vi "Continuous DO Output.vi"() -> ()   [LabVIEW 2016]
uses:
  <vilib>/ULx/Create Channel.llb/ULx Create Channel (AI-Voltage-Basic).vi
  <vilib>/ULx/Timing.llb/ULx Timing (Sample Clock).vi
  <vilib>/ULx/Read.llb/ULx Read (Analog 1D Wfm NChan NSamp).vi
  <vilib>/Waveform/WDTOps.llb/WDT Index Channel DBL.vi
panel:
  in  "Boolean 3":bool
  out "Waveform Graph":dbl[](graph)
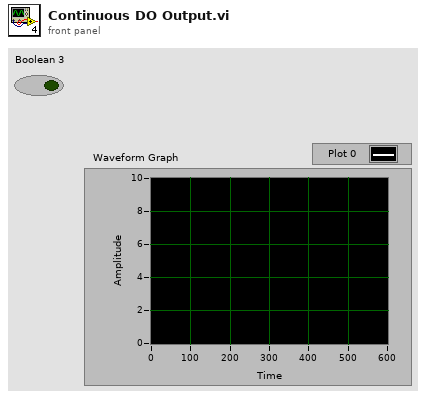
[diagram p1: front panel]
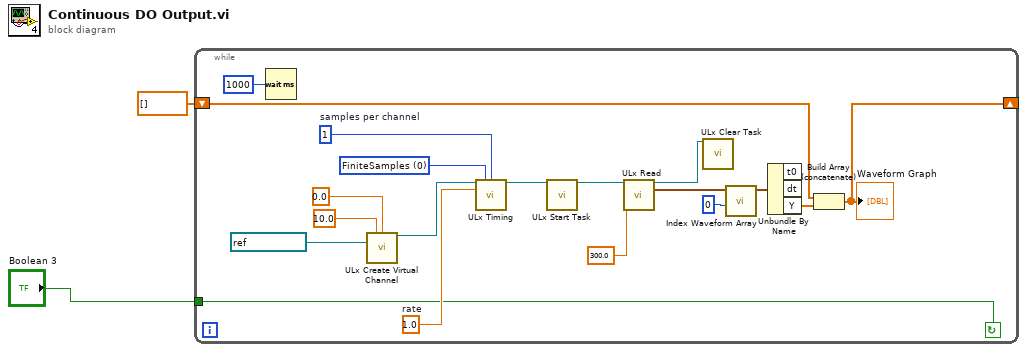
[diagram p0: block diagram]
diagram:
  n1 = while {
    shift-right: [w5] -> _
    shift-left: dbl[] [] -> [w7]
    tunnel: "Boolean 3" -> [w3]
    stop <- w3 continue-if-true
    w6 = 1  # samples per channel
    w17 = 0 items=["FiniteSamples", "ContinuousSamples"] ("sample mode")
    w16 = 1.0  # rate
    n2 = Wait (ms)(milliseconds to wait=u32 1000) -> ()  [unwired: 1 out]
    n3 = call-poly <vilib>:"ULx Create Virtual Channel.vi"("maximum value"=10.0, "minimum value"=0.0, "physical channels"=refnum<k21> "Dev0/Ai0" ("Test 1")) -> ("task out"=w14:refnum<k24>)  [unwired: 11 in, 1 out]
    n4 = call-poly <vilib>:"ULx Timing.vi"("task in"=w14, "sample mode"=w17, "samples per channel"=w6, "rate"=w16) -> ("task out"=w15:refnum<k24>)  [unwired: 10 in, 1 out]
    n5 = call <vilib>:"ULx Start Task.vi"("task in"=w15) -> ("task out"=w18:refnum<k24>)  [unwired: 13 in, 1 out]
    n6 = call-poly <vilib>:"ULx Read.vi"("task in"=w18, "timeout"=300.0) -> ("task out"=w11:refnum<k24>, "data"=w21:waveform(dbl)[])  [unwired: 11 in, 1 out]
    n7 = call <vilib>:"ULx Clear Task.vi"("task in"=w11) -> ()  [unwired: 14 in, 1 out]
    n8 = call-poly <vilib>:"Index Waveform Array.vi"("index"=0, "waveform array"=w21) -> ("waveform"=w20:waveform(dbl))  [unwired: 8 in, 1 out]
    n9 = Unbundle By Name(w20) -> ("Y"=w9:dbl[])  [unwired: 2 out]
    n10 = Build Array (concatenate)(w7, w9) -> (w5:dbl[])
    "Waveform Graph" <- w5
  }
